vi "_DEPRICATED FRCts20_WebMethods_Notifications_PUT.vi"() -> ()   [LabVIEW 2014, in "FRCts20_WebMethods.lvlib"]
uses:
  FRCts20_WebMethods.lvlib
  <vilib>/wsapi/NI_WebServices.lvlib
  Backend/source/VI Source/FRCts20_Backend_API/FRCts20_Backend_API_EventRoot.vi
  Backend/source/VI Source/FRCts20_Backend_API/FRCts20_Backend_API_Command_EventRoot.ctl
  FRCts20_WebMethods_Redirect_Team.vi
  Backend/source/VI Source/FRCts20_Backend_API/FRCts20_Backend_API_EventRoot.ctl
panel:
  out "EventRoot Out":T1
  in  "httpRequestID":u32
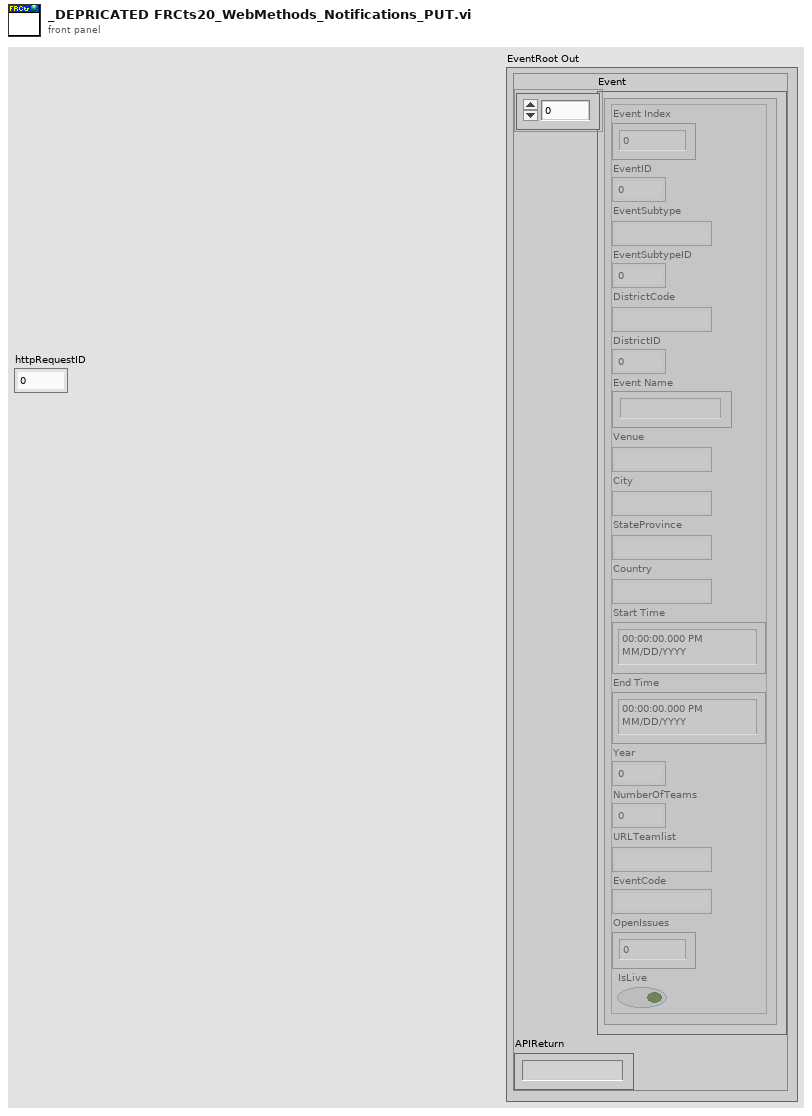
[diagram p1: front panel]
types:
  T1 = typedef "FRCts20_Backend_API.lvlib/FRCts20_Backend_API_EventRoot.ctl" = cluster{"Event":cluster{"Event Index":u32, "EventID":u32, "EventSubtype":string, "EventSubtypeID":u32, "DistrictCode":string, "DistrictID":u32, "Event Name":string, "Venue":string, "City":string, "StateProvince":string, "Country":string, "Start Time":timestamp, "End Time":timestamp, "Year":u32, "NumberOfTeams":u32, "URLTeamlist":string, "EventCode":string, "OpenIssues":u8, "IsLive":bool}[], "APIReturn":string}
  T2 = typedef "FRCts20_Backend_API.lvlib/FRCts20_Backend_API_Command_EventRoot.ctl" = string
  T3 = cluster{"Event Index":u32, "EventID":u32, "EventSubtype":string, "EventSubtypeID":u32, "DistrictCode":string, "DistrictID":u32, "Event Name":string, "Venue":string, "City":string, "StateProvince":string, "Country":string, "Start Time":timestamp, "End Time":timestamp, "Year":u32, "NumberOfTeams":u32, "URLTeamlist":string, "EventCode":string, "OpenIssues":u8, "IsLive":bool}[]
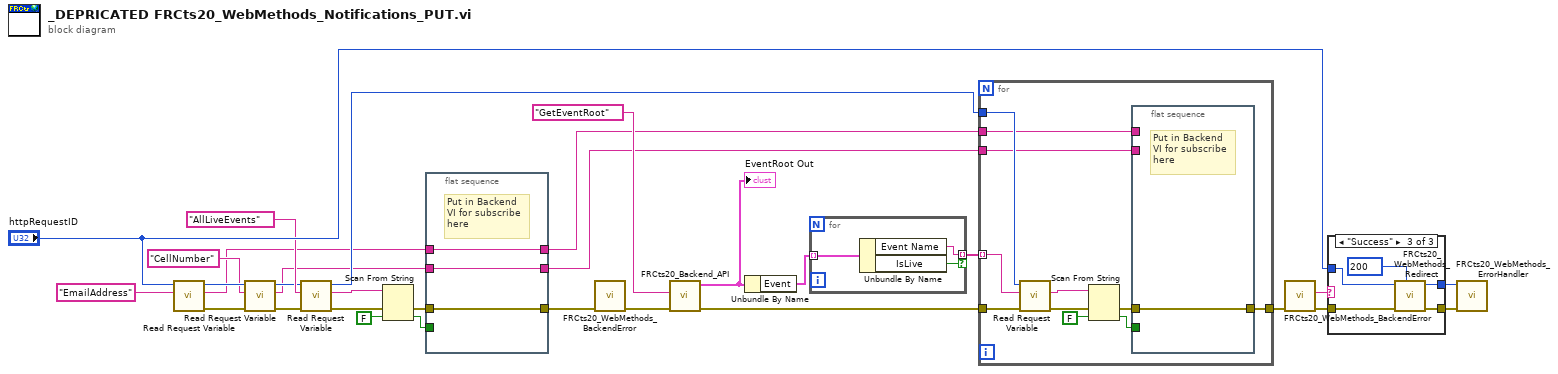
[diagram p0: block diagram]
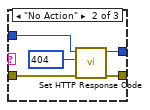
[diagram p3: hidden frame]
diagram:
  n1 = call <vilib>:"Read Request Variable.vi"("variable name"="EmailAddress", "httpRequestID"="httpRequestID") -> ("error out"=w24:errorcluster, "value"=w7:string, "httpRequestID out"=w23:u32)  [unwired: 7 in]
  n2 = call <vilib>:"Read Request Variable.vi"("error in (no error)"=w24, "variable name"="CellNumber", "httpRequestID"=w23) -> ("error out"=w20:errorcluster, "value"=w8:string, "httpRequestID out"=w11:u32)  [unwired: 6 in]
  n3 = call <vilib>:"Read Request Variable.vi"("error in (no error)"=w20, "variable name"="AllLiveEvents", "httpRequestID"=w11) -> ("error out"=w19:errorcluster, "value"=w17:string, "httpRequestID out"=w12:u32)  [unwired: 6 in]
  n4 = Scan From String(input string=w17, error in=w19, default 1=FALSE) -> (error out=w10:errorcluster, output 1=w9:bool)  [unwired: 2 in, 2 out]
  n5 = flat-sequence {
    tunnel: [w33] -> w2
    tunnel: w10 -> [w33]
    tunnel: w9 -> [_]
    tunnel: w8 -> [w32]
    tunnel: w7 -> [w31]
    tunnel: [w32] -> w6
    tunnel: [w31] -> w5
    frame #0 {
      # "Put in Backend VI for subscribe here"
    }
  }
  n6 = call "FRCts20_WebMethods_BackendError.vi"("error in (no error)"=w2) -> ("error out"=w1:errorcluster)  [unwired: 9 in, 1 out]
  n7 = call-poly "FRCts20_Backend_API.vi"("error in (no error)"=w1, "Message"=T2 "GetEventRoot") -> ("error out"=w3:errorcluster, "EventRoot Out"=w15:T1)  [unwired: 7 in, 1 out]
  "EventRoot Out" <- w15
  n8 = Unbundle By Name(w15) -> ("Event"=w14:T3)
  n9 = for {
    tunnel: w14 -> [w36] mode=indexing
    tunnel: [w35] -> w13 mode=indexing if=w34
    n10 = Unbundle By Name(w36) -> ("Event Name"=w35:string, "IsLive"=w34:bool)
  }
  n11 = for {
    tunnel: w13 -> [w47] mode=indexing
    tunnel: w12 -> [w46]
    tunnel: w3 -> [w40]
    tunnel: w6 -> [w39]
    tunnel: w5 -> [w38]
    tunnel: [w37] -> w4
    n12 = call <vilib>:"Read Request Variable.vi"("error in (no error)"=w40, "variable name"=w47, "httpRequestID"=w46) -> ("error out"=w44:errorcluster, "value"=w45:string)  [unwired: 6 in, 1 out]
    n13 = Scan From String(input string=w45, error in=w44, default 1=FALSE) -> (error out=w42:errorcluster, output 1=w41:bool)  [unwired: 2 in, 2 out]
    n14 = flat-sequence {
      tunnel: [w48] -> w37
      tunnel: w42 -> [w48]
      tunnel: w41 -> [_]
      tunnel: w39 -> [_]
      tunnel: w38 -> [_]
      frame #0 {
        # "Put in Backend VI for subscribe here"
      }
    }
  }
  n15 = call "FRCts20_WebMethods_BackendError.vi"("error in (no error)"=w4) -> ("error out"=w27:errorcluster, "Status out"=w26:string)  [unwired: 9 in]
  n16 = case shown="\"Success\"" w26 {
    tunnel: [w50 w55 w60] -> w29
    tunnel: [w49 w54 w59] -> w30
    tunnel: w27 -> [w50 w52 w58]
    tunnel: "httpRequestID" -> [w49 w53 w57]
    frame "Backend Error", Default {
    }
    frame "No Action" {
      w51 = 404 items=["100"=100, "101"=101, "200"=200, "201"=201, "202"=202, "203"=203, "204"=204, "205"=205, "206"=206, "300"=300, "301"=301, "302"=302, "303"=303, "304"=304, "305"=305, "306"=306, "307"=307, "400"=400, "401"=401, "402"=402, "403"=403, "404"=404, "405"=405, "406"=406, "407"=407, "408"=408, "409"=409, "410"=410, "411"=411, "412"=412, "413"=413, "414"=414, "415"=415, "416"=416, "417"=417, "500"=500, "501"=501, "502"=502, "503"=503, "504"=504, "505"=505] ("response code (200)")
      n17 = call <vilib>:"Set HTTP Response Code.vi"("error in (no error)"=w52, "response code (200)"=w51, "httpRequestID"=w53) -> ("error out"=w55:errorcluster, "httpRequestID out"=w54:u32)  [unwired: 7 in]
    }
    frame "Success" {
      w56 = 200 items=["100"=100, "101"=101, "200"=200, "201"=201, "202"=202, "203"=203, "204"=204, "205"=205, "206"=206, "300"=300, "301"=301, "302"=302, "303"=303, "304"=304, "305"=305, "306"=306, "307"=307, "400"=400, "401"=401, "402"=402, "403"=403, "404"=404, "405"=405, "406"=406, "407"=407, "408"=408, "409"=409, "410"=410, "411"=411, "412"=412, "413"=413, "414"=414, "415"=415, "416"=416, "417"=417, "500"=500, "501"=501, "502"=502, "503"=503, "504"=504, "505"=505] ("response code (200)")
      n18 = call-poly "FRCts20_WebMethods_Redirect.vi"("response code (200)"=w56, "error in (no error)"=w58, "httpRequestID"=w57) -> ("error out"=w60:errorcluster, "httpRequestID out"=w59:u32)  [unwired: 7 in]
    }
  }
  n19 = call "FRCts20_WebMethods_ErrorHandler.vi"("error in"=w29, "LabVIEW Web Service Request"=w30) -> ()  [unwired: 8 in, 2 out]
